vi "XML.Sequences.ListActive.vi"(8 "error in":errorcluster, 11 "XML file path":path) -> (0 "error out":errorcluster, 2 "values":string[](array[string]))   [LabVIEW 2019, in "Tools.lvlib"]
uses:
  Tools.lvlib
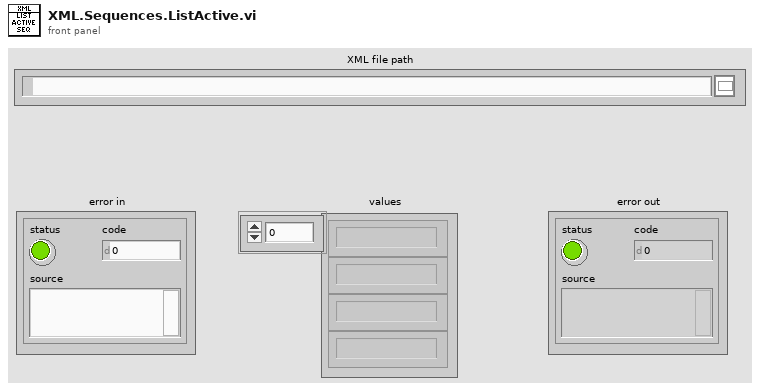
[diagram p1: front panel]
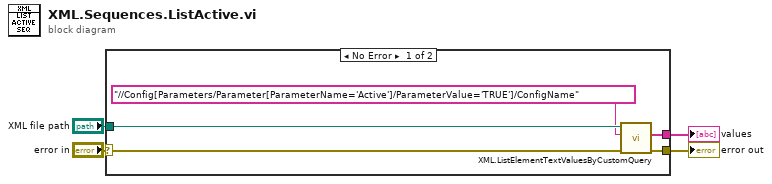
[diagram p0: block diagram]
diagram:
  n1 = case shown="No Error" "error in" {
    selector: "error in" -> [w8 w10]
    tunnel: [w7 w10] -> w4
    tunnel: "XML file path" -> [w9 _]
    tunnel: [w6 _] -> w1
    frame No Error {
      n2 = call "XML.ListElementTextValuesByCustomQuery.vi"("error in"=w8, "XPath expression"="//Config[Parameters/Parameter[ParameterName='Active']/ParameterValue='TRUE']/ConfigName", "XML file path"=w9) -> ("error out"=w7:errorcluster, "values"=w6:string[])  [unwired: 7 in]
    }
    frame Error {
    }
  }
  "error out" <- w4
  "values" <- w1
